vi "Enable Trigger Averaging.vi"(7 "Enable Averaging Trigger Function (F: Disable)":bool, 8 "error in (no error)":errorcluster, 11 "VISA resource name":refnum<visa-resource-name>) -> (0 "error out":errorcluster, 3 "VISA resource name out":refnum<visa-resource-name>)   [LabVIEW 2022 SP3, in "Agilent ENA Series.lvlib"]
doc: "Configures the averaging trigger function.\n\nNote: \nThe VI is not supported when TRIG:SEQ:SOUR is INTernal or EXTernal in <b>Configure Trigger.Vi</b>"
uses:
  <instrlib>/Agilent ENA Series/Agilent ENA Series.lvlib
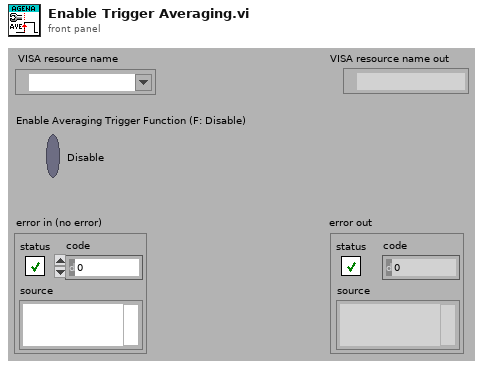
[diagram p1: front panel]
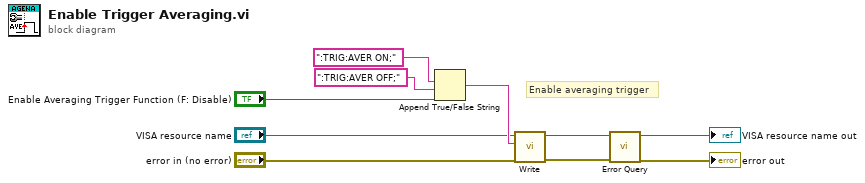
[diagram p0: block diagram]
diagram:
  # "Enable averaging trigger"
  n1 = Append True/False String(1:"Enable Averaging Trigger Function (F: Disable)", 2:":TRIG:AVER OFF;", 3:":TRIG:AVER ON;") -> (0:w5:string)  [unwired: 1 out]
  n2 = call <instrlib>:"Write.vi"("error in (no error)"="error in (no error)", "String ()"=w5, "VISA resource name"="VISA resource name") -> ("error out"=w1:errorcluster, "VISA resource name out"=w2:refnum<visa-resource-name>)  [unwired: 6 in, 1 out]
  n3 = call <instrlib>:"Error Query.vi"("error in (no error)"=w1, "VISA resource name"=w2) -> ("error out"=→"error out":errorcluster, "VISA resource name out"=→"VISA resource name out":refnum<visa-resource-name>)  [unwired: 8 out]
